vi "Byte Buffer.Write (I8).vi"(8 "error in (no error)":errorcluster, 9 "value":i8, 10 "buffer offset":u64, 11 "Byte Buffer in":refnum<class "Byte Buffer.lvclass">) -> (0 "error out":errorcluster, 3 "Byte Buffer out":refnum<class "Byte Buffer.lvclass">)   [LabVIEW 2016, in "VeriStand Data.lvlib" / "Byte Buffer.lvclass"]
doc: "Writes <B>value</B> to the provided <B>Byte Buffer</B> at location <B>buffer offset</B> in the format of the data type specified."
uses:
  Byte Buffer.lvclass
  Byte Buffer.lvclass/Byte Buffer.ctl
  Byte Buffer.Write (String).vi
  Byte Buffer.Buffer Subset.Set.vi
  Memory Management/Memory Management.MoveByteBlock.Read (String).vi
  Memory Management/Memory Management.Handle Return.vi
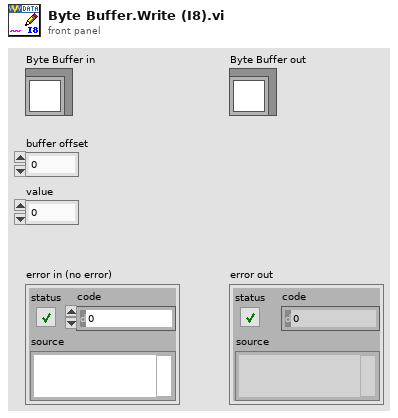
[diagram p1: front panel]
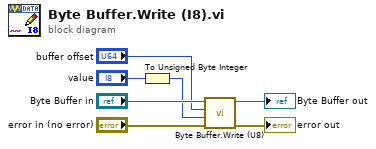
[diagram p0: block diagram]
diagram:
  n1 = To Unsigned Byte Integer(number="value") -> (unsigned 8bit integer=w1:u8)
  n2 = call "Byte Buffer.Write (U8).vi"("error in (no error)"="error in (no error)", "value"=w1, "buffer offset"="buffer offset", "Byte Buffer in"="Byte Buffer in") -> ("error out"=→"error out":errorcluster, "Byte Buffer out"=→"Byte Buffer out":refnum<class "Byte Buffer.lvclass">)  [unwired: 6 in]
